vi "read_msg_to_log.vi"(10 "string_type (csv)":enum16{"none", "csv", "json", "xml"}(ring)=enum."csv", 11 "Error in":refnum<class "Error.lvclass">) -> (2 "error_msg_to_log":string)   [LabVIEW 2023, in "Error Handling Interface.lvlib" / "Error.lvclass"]
doc: "Returns the message to <B>log</B>"
uses:
  Error.lvclass
  Error.lvclass/Error.ctl
  <vilib>/JDP Science/JSONtext/Variant to JSON Text.vi
  <vilib>/JDP Science/JSONtext/LVClass Serializer/JSONtext LVClass Serializer.lvclass
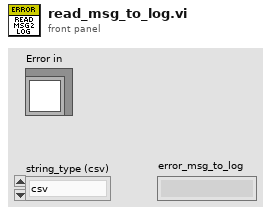
[diagram p1: front panel]
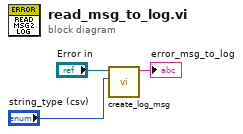
[diagram p0: block diagram]
diagram:
  n1 = call "create_log_msg.vi"("string_type"="string_type (csv)", "Error in"="Error in") -> ("error_msg_to_log"=→"error_msg_to_log":string)  [unwired: 9 in]
